vi "Simple Single Task.vi"(9 "B":dbl, 10 "A":dbl, 11 "Promise":refnum<class "Promise.lvclass">) -> ()   [LabVIEW 2020, in "Futures-Examples.lvlib"]
uses:
  Futures-Examples.lvlib
  0cc008d6-47af-4b6a-9da6-3fd1db2280fb.vi
  Promises/Promise/Promise.lvclass
  DoubleValue/DoubleValue.lvclass
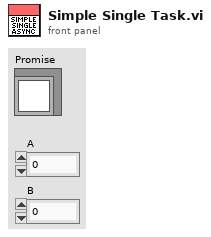
[diagram p1: front panel]
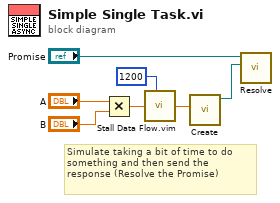
[diagram p0: block diagram]
diagram:
  # "Simulate taking a bit of time to do something and then send the response (Resolve the Promise)"
  n1 = Multiply(x="A", y="B") -> (x*y=w5:dbl)
  n2 = call "Stall Data Flow.vim"("value in"=w5, "milliseconds to wait"=u32 1200) -> ("value out"=w3:dbl)  [unwired: 1 out]
  n3 = call "Create.vi"("Value"=w3) -> ("DoubleValue"=w2:refnum<class "DoubleValue.lvclass">)  [unwired: 10 in]
  n4 = call "Resolve.vi"("Result"=w2, "Promise in"="Promise") -> ()  [unwired: 8 in, 2 out]
